vi "2tdms.vi"() -> ()   [LabVIEW 2010]
panel:
  in  "Dateiordner":path=path "C:/Users/Atmos/Desktop/Johnny"
  out "nächste TDMS-Datei":refnum<k34>
  out "aktuelle TDMS-Datei":refnum<k34>
  out "Zyklusnummer":u32
  out "Wert":i32
  out "Zykluszeit":u32
  in  "Zykluslänge":u32
  out "Anzeige":u32
  out "Zeit":u32
  in  "Stopp":bool
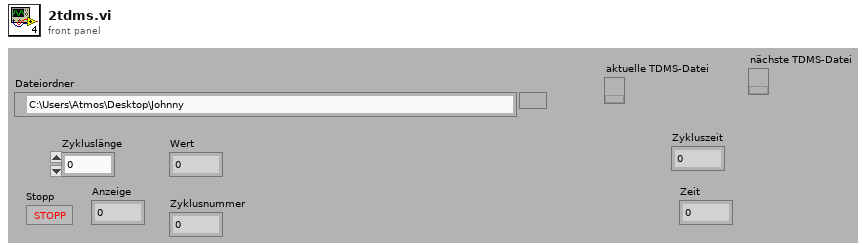
[diagram p1: front panel]
types:
  T1 = enum16{"open", "open or create", "create or replace", "create", "open (read-only)"}
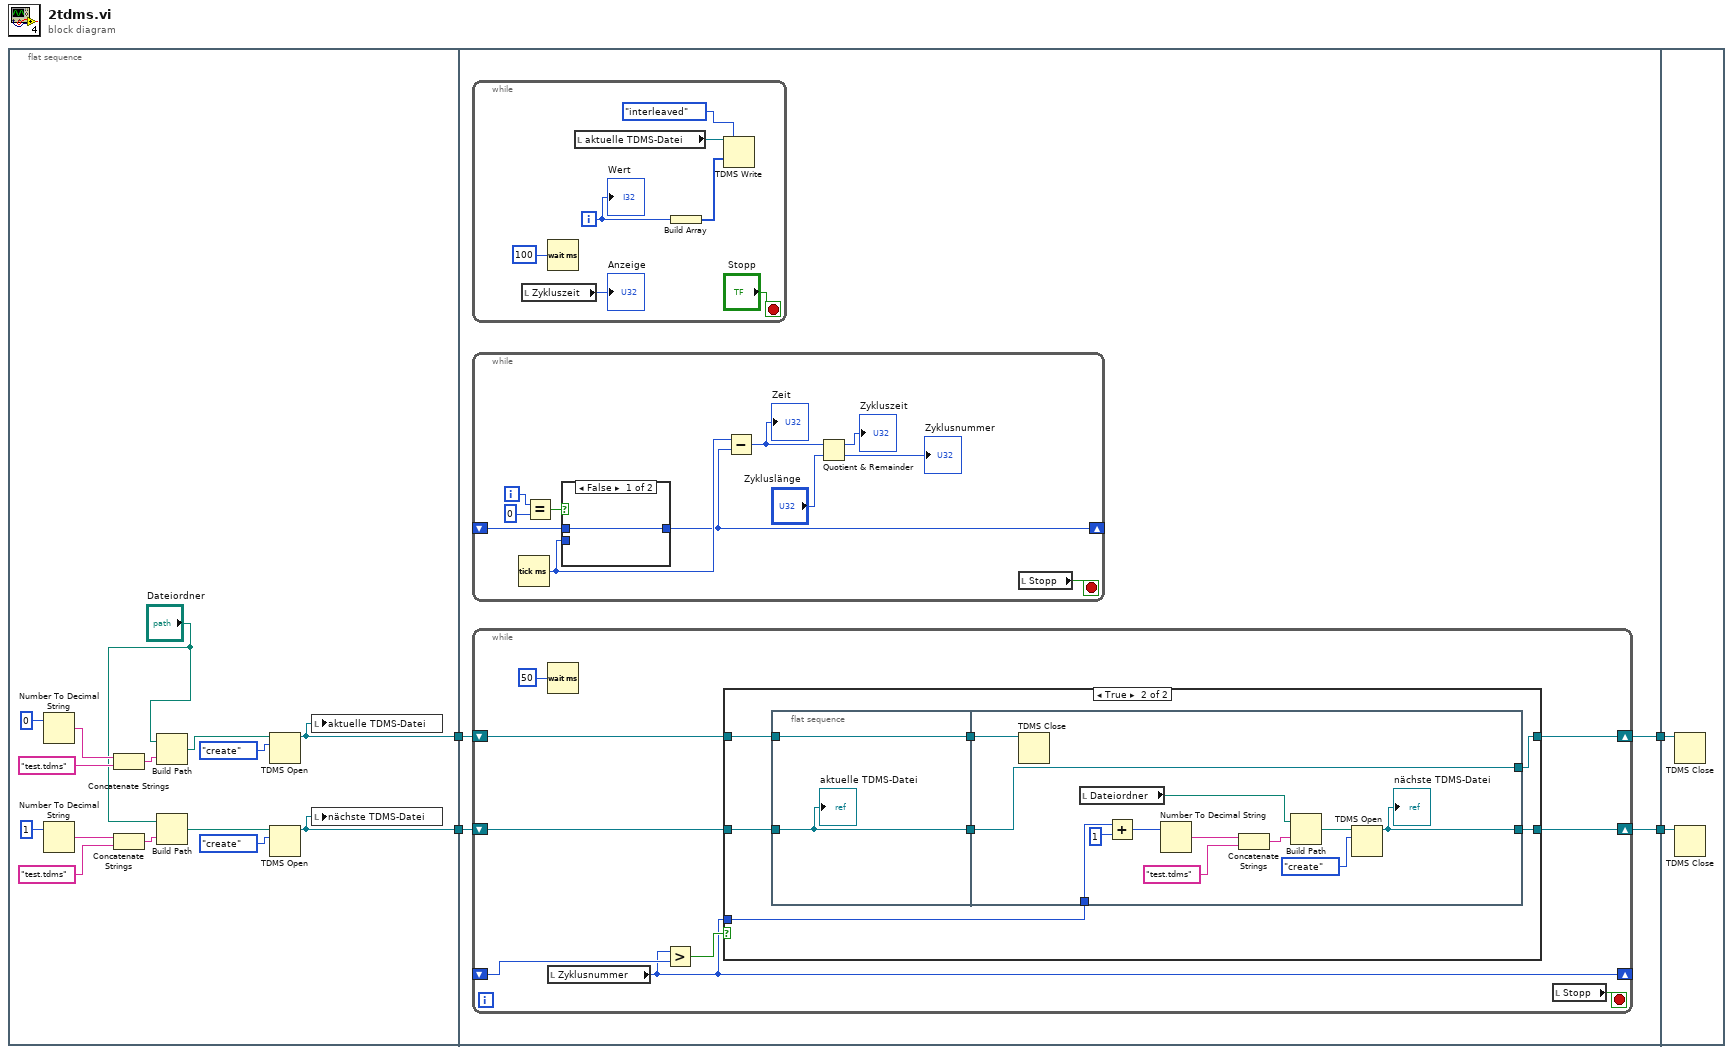
[diagram p0: block diagram]
diagram:
  n1 = flat-sequence {
    tunnel: [w7] -> w4
    tunnel: [w6] -> w3
    tunnel: w4 -> [w23]
    tunnel: w3 -> [w22]
    tunnel: [w21] -> w2
    tunnel: [w20] -> w1
    tunnel: w2 -> [w77]
    tunnel: w1 -> [w76]
    frame #0 {
      n2 = Number To Decimal String(number=0 ("Wert")) -> (decimal integer string=w17:string)  [unwired: 1 in]
      n3 = Number To Decimal String(number=1 ("Wert")) -> (decimal integer string=w12:string)  [unwired: 1 in]
      n4 = Concatenate Strings(w17, "test.tdms" ("String")) -> (w15:string)
      n5 = Concatenate Strings(w12, "test.tdms" ("String")) -> (w10:string)
      n6 = Build Path(base path="Dateiordner", name or relative path=w15) -> (appended path=w18:path)
      n7 = Build Path(base path="Dateiordner", name or relative path=w10) -> (appended path=w13:path)
      n8 = TDMS Open(10:T1."create" ("Operation (0:Öffnen)"), 11:w18) -> (3:w7:refnum<k34>)  [unwired: 4 in, 1 out]
      n9 = TDMS Open(10:T1."create" ("Operation (0:Öffnen)"), 11:w13) -> (3:w6:refnum<k34>)  [unwired: 4 in, 1 out]
      n10 = local write "aktuelle TDMS-Datei"(w7) -> ()
      n11 = local write "nächste TDMS-Datei"(w6) -> ()
    }
    frame #1 {
      n12 = while {
        i -> [w71]
        stop <- "Stopp" stop-if-true
        n13 = local read "Zykluszeit"() -> (→"Anzeige":u32)
        n14 = Wait (ms)(milliseconds to wait=u32 100 ("Zu wartende ms")) -> ()  [unwired: 1 out]
        n15 = local read "aktuelle TDMS-Datei"() -> (w69:refnum<k34>)
        n16 = Build Array(w71) -> (w70:i32[])
        n17 = TDMS Write(0:w69, 1:enum16{"decimated", "interleaved"}."interleaved" ("Daten-Layout (0:dezimiert)"), 9:w70) -> ()  [unwired: 3 in, 4 out]
        "Wert" <- w71
      }
      n18 = while {
        shift-right: [w60] -> _
        shift-left: _ -> [w62]
        i -> [w65]
        stop <- w66 stop-if-true
        n19 = Tick Count (ms)() -> (millisecond timer value=w61:u32)
        n20 = Equal?(x=w65, y=0) -> (x = y?=w63:bool)
        n21 = case shown="False" w63 {
          tunnel: w61 -> [_ w68]
          tunnel: [w67 w68] -> w60
          tunnel: w62 -> [w67 _]
          frame False {
          }
          frame True {
          }
        }
        n22 = Subtract(x=w61, y=w60) -> (x-y=w59:u32)
        "Zeit" <- w59
        n23 = Quotient & Remainder(x=w59, y="Zykluslänge") -> (x-y*floor(x/y)=→"Zykluszeit":u32, floor(x/y)=→"Zyklusnummer":u32)
        n24 = local read "Stopp"() -> (w66:bool)
      }
      n25 = while {
        shift-right: [w28] -> _
        shift-left: _ -> [w30]
        shift-right: [w25] -> w21
        shift-left: w22 -> [w26]
        shift-right: [w24] -> w20
        shift-left: w23 -> [w27]
        stop <- w31 stop-if-true
        n26 = Wait (ms)(milliseconds to wait=u32 50 ("Zu wartende ms")) -> ()  [unwired: 1 out]
        n27 = local read "Zyklusnummer"() -> (w28:u32)
        n28 = Greater?(x=w28, y=w30) -> (0:w29:bool)
        n29 = case shown="True" w29 {
          tunnel: w28 -> [_ w35]
          tunnel: [w34 w36] -> w24
          tunnel: w27 -> [w34 w39]
          tunnel: [w33 w41] -> w25
          tunnel: w26 -> [w33 w40]
          frame False {
          }
          frame True {
            n30 = flat-sequence {
              tunnel: w40 -> [w43]
              tunnel: w39 -> [w42]
              tunnel: [w43] -> w38
              tunnel: [w42] -> w37
              tunnel: [w48] -> w41
              tunnel: w38 -> [w47]
              tunnel: w37 -> [w46]
              tunnel: [w47] -> w36
              tunnel: w35 -> [w45]
              frame #0 {
                "aktuelle TDMS-Datei" <- w43
              }
              frame #1 {
                n31 = TDMS Close(11:w46) -> ()  [unwired: 1 in, 2 out]
                n32 = local read "Dateiordner"() -> (w44:path)
                n33 = Add(x=w45, y=u32 1) -> (x+y=w53:u32)
                n34 = Number To Decimal String(number=w53) -> (decimal integer string=w51:string)  [unwired: 1 in]
                n35 = Concatenate Strings(w51, "test.tdms" ("String")) -> (w49:string)
                n36 = Build Path(base path=w44, name or relative path=w49) -> (appended path=w54:path)
                n37 = TDMS Open(10:T1."create" ("Operation (0:Öffnen)"), 11:w54) -> (3:w48:refnum<k34>)  [unwired: 4 in, 1 out]
                "nächste TDMS-Datei" <- w48
              }
            }
          }
        }
        n38 = local read "Stopp"() -> (w31:bool)
      }
    }
    frame #2 {
      n39 = TDMS Close(11:w76) -> ()  [unwired: 1 in, 2 out]
      n40 = TDMS Close(11:w77) -> ()  [unwired: 1 in, 2 out]
    }
  }
